vi "myXi_AcquireImage.vi"(8 "error in":errorcluster, 10 "acquisition frame":T1, 11 "xiCam In":refnum<k24>) -> (0 "error out":errorcluster, 2 "acquisition frame out":T1, 3 "xiCam Out":refnum<k24>, 4 "no Frame Dropped":bool, 6 "time for acquire":dbl[unit])   [LabVIEW 2018]
uses:
  C:/XIMEA/API/x64/xiApi.NETX64.dll
  typedef/AcquisitionFrame.ctl
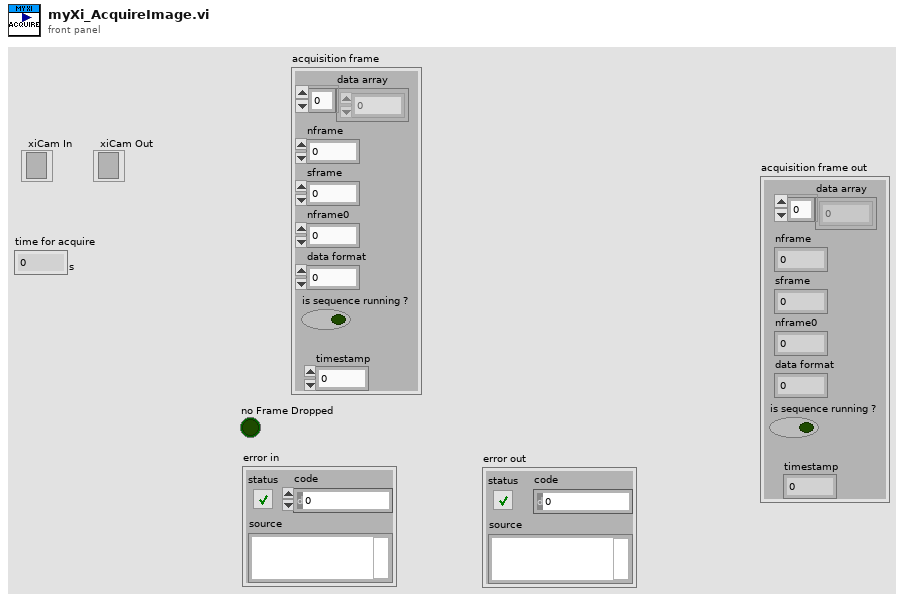
[diagram p1: front panel]
types:
  T1 = typedef "AcquisitionFrame.ctl" = cluster{"data array":u8[], "nframe":i32, "sframe":i32, "nframe0":i32, "data format":i32, "is sequence running ?":bool, "timestamp":dbl}
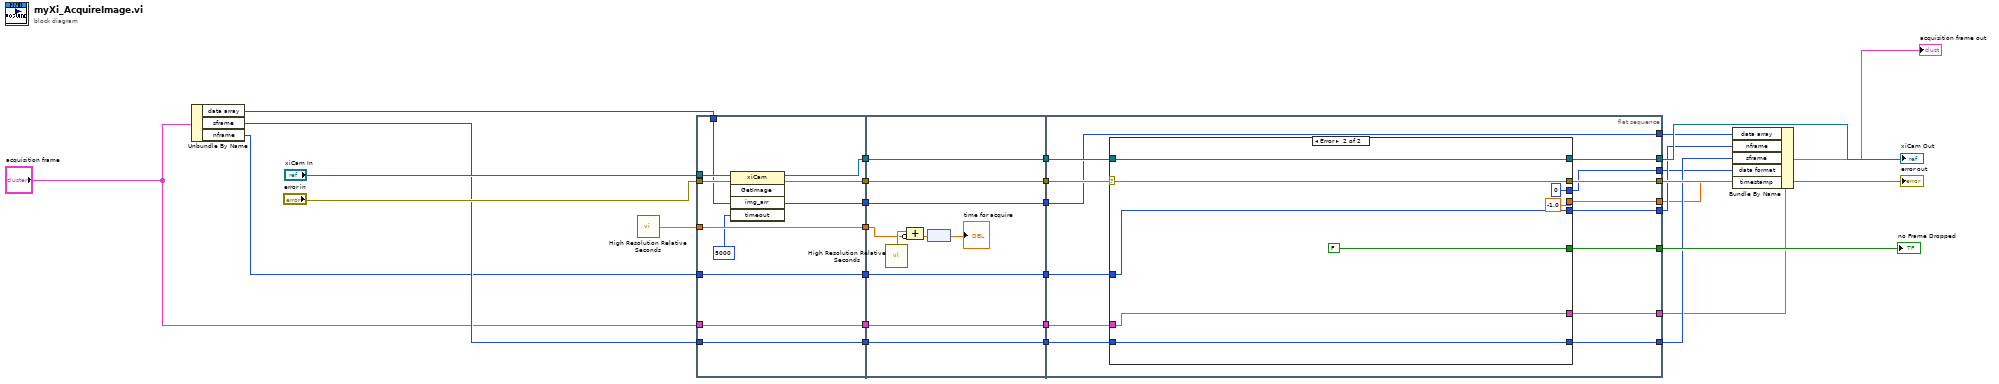
[diagram p0: block diagram]
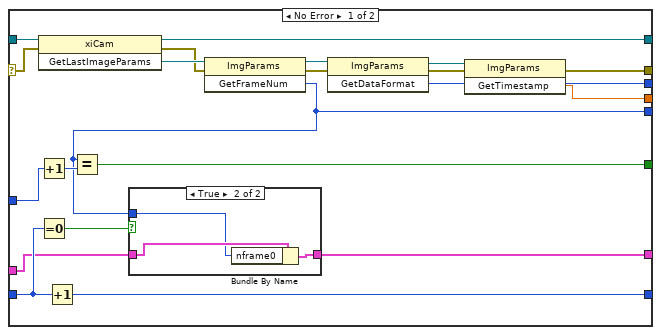
[diagram p2: hidden frame]
diagram:
  n1 = Unbundle By Name("acquisition frame") -> ("data array"=w17:u8[], "sframe"=w14:i32, "nframe"=w10:i32)
  n2 = call <vilib>:"High Resolution Relative Seconds.vi"() -> ("relative seconds"=w24:dbl)
  n3 = flat-sequence {
    tunnel: "xiCam In" -> [w40]
    tunnel: w17 -> [w31]
    tunnel: "error in" -> [w36]
    tunnel: w24 -> [w41]
    tunnel: [w39] -> w30
    tunnel: [w38] -> w29
    tunnel: [w35] -> w28
    tunnel: [w41] -> w27
    tunnel: w14 -> [w34]
    tunnel: [w34] -> w12
    tunnel: w10 -> [w33]
    tunnel: [w33] -> w8
    tunnel: "acquisition frame" -> [w32]
    tunnel: [w32] -> w6
    tunnel: w30 -> [w51]
    tunnel: w29 -> [w50]
    tunnel: w28 -> [w49]
    tunnel: w27 -> [w46]
    tunnel: [w51] -> w23
    tunnel: [w50] -> w22
    tunnel: [w49] -> w21
    tunnel: [w44] -> w13
    tunnel: w12 -> [w44]
    tunnel: [w43] -> w9
    tunnel: w8 -> [w43]
    tunnel: [w42] -> w7
    tunnel: w6 -> [w42]
    tunnel: w23 -> [w64]
    tunnel: w22 -> [w59]
    tunnel: w21 -> [w65]
    tunnel: [w63] -> w20
    tunnel: [w62] -> w15
    tunnel: [w61] -> w19
    tunnel: [w60] -> w18
    tunnel: [w59] -> w16
    tunnel: w13 -> [w58]
    tunnel: [w57] -> w11
    tunnel: w9 -> [w56]
    tunnel: w7 -> [w55]
    tunnel: [w54] -> w5
    tunnel: [w53] -> w4
    tunnel: [w52] -> w1
    frame #0 {
      n4 = invoke class="xiCam" method="GetImage"(reference=w40, error in=w36, "img_arr"=w31, "timeout"=5000) -> (reference out=w39:refnum<k24>, error out=w35:errorcluster, "img_arr"=w38:u8[])  [unwired: 1 in, 2 out]
    }
    frame #1 {
      n5 = call <vilib>:"High Resolution Relative Seconds.vi"() -> ("relative seconds"=w47:dbl)
      n6 = Compound Arithmetic op=ADD(w47, invert w46) -> (w48:dbl)
      n7 = node(w48) -> (→"time for acquire":dbl[unit])
    }
    frame #2 {
      n8 = case shown="Error" w65 {
        selector: w65 -> [w80 w95]
        tunnel: w64 -> [w85 w97]
        tunnel: [w84 w97] -> w63
        tunnel: [w74 w92] -> w62
        tunnel: [w81 FALSE] -> w61
        tunnel: [w69 w95] -> w60
        tunnel: w58 -> [w76 w94]
        tunnel: [w78 w94] -> w57
        tunnel: w56 -> [w75 w92]
        tunnel: w55 -> [w73 w93]
        tunnel: [w72 w93] -> w54
        tunnel: [w68 0 ("GetDataFormat")] -> w53
        tunnel: [w66 -1.0 ("GetTimestamp")] -> w52
        frame No Error {
          n9 = invoke class="xiCam" method="GetLastImageParams"(reference=w85, error in=w80) -> (reference out=w84:refnum<k24>, error out=w79:errorcluster, "GetLastImageParams"=w83:refnum<k24>)  [unwired: 1 in]
          n10 = Increment(x=w75) -> (x+1=w82:i32)
          n11 = Equal To 0?(x=w76) -> (x = 0?=w77:bool)
          n12 = Increment(x=w76) -> (x+1=w78:i32)
          n13 = invoke class="ImgParams" method="GetFrameNum"(reference=w83, error in=w79) -> (reference out=w70:refnum<k24>, error out=w71:errorcluster, "GetFrameNum"=w74:i32)  [unwired: 1 in]
          n14 = Equal?(x=w74, y=w82) -> (x = y?=w81:bool)
          n15 = case shown="True" w77 {
            tunnel: w74 -> [_ w88]
            tunnel: w73 -> [w86 w89]
            tunnel: [w86 w87] -> w72
            frame False {
            }
            frame True {
              n16 = Bundle By Name(cluster=w89, "nframe0"=w88) -> (w87:T1)
            }
          }
          n17 = invoke class="ImgParams" method="GetDataFormat"(reference=w70, error in=w71) -> (reference out=w67:refnum<k24>, error out=w69:errorcluster, "GetDataFormat"=w68:i32)  [unwired: 1 in]
          n18 = invoke class="ImgParams" method="GetTimestamp"(reference=w67) -> ("GetTimestamp"=w66:dbl)  [unwired: 2 in, 2 out]
        }
        frame Error {
        }
      }
    }
  }
  n19 = Bundle By Name(cluster=w5, "data array"=w16, "nframe"=w15, "sframe"=w11, "data format"=w4, "timestamp"=w1) -> (→"acquisition frame out":T1)
  "xiCam Out" <- w20
  "error out" <- w18
  "no Frame Dropped" <- w19
